vi "Read Configuration Parameters.vi"(8 "error in (no error)":errorcluster, 10 "refnum":T1, 11 "HW Configuration in":refnum<class "HW Configuration.lvclass">) -> (0 "error out":errorcluster, 2 "refnum out":T1, 3 "HW Configuration out":refnum<class "HW Configuration.lvclass">)   [LabVIEW 2017, in "Hardware.lvlib" / "HW Configuration.lvclass"]
uses:
  HW Configuration.lvclass
  C:/Program Files (x86)/National Instruments/LabVIEW 2017/user.lib/Configuration Dialog Actor/Configuration.lvclass
  <vilib>/Utility/config.llb/Config Data RefNum.ctl
  <userlib>/Configuration Dialog Actor/Configuration.lvclass/Configuration.ctl
  HW Configuration.lvclass/HW Configuration.ctl
  <userlib>/Configuration Dialog Actor/Configuration.lvclass
  <vilib>/Utility/config.llb/NI_LVConfig.lvlib
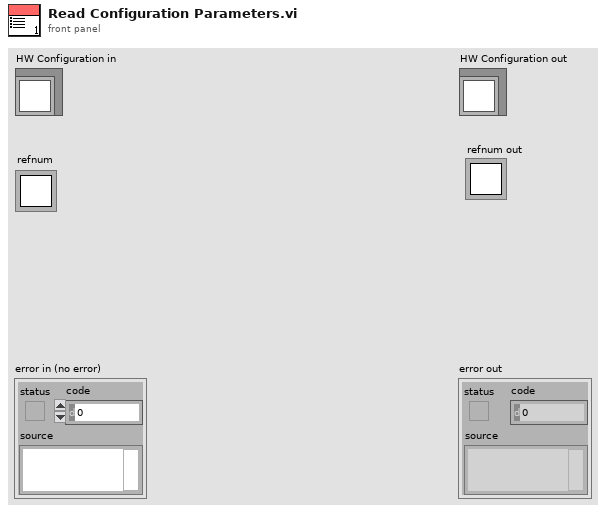
[diagram p1: front panel]
types:
  T1 = typedef "NI_LVConfig.lvlib/Config Data RefNum.ctl" = refnum<k1>
  T2 = cluster{"Device Name":string, "Channel Mapping (Device -> Channel)":string[][]}
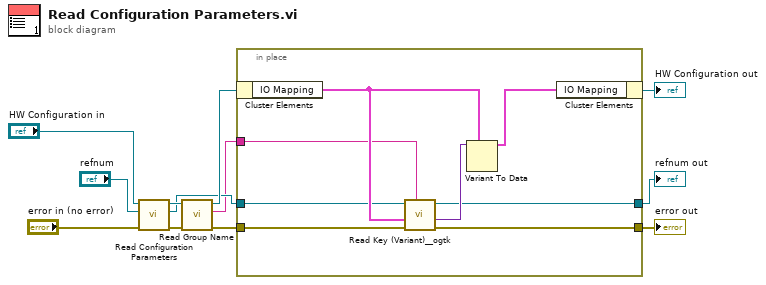
[diagram p0: block diagram]
diagram:
  n1 = call-parent "Read Configuration Parameters.vi"("error in (no error)"="error in (no error)", "refnum"="refnum", "Configuration in"="HW Configuration in") -> ("error out"=w6:errorcluster, "refnum out"=w7:T1, "Configuration out"=w9:refnum<class "HW Configuration.lvclass">)  [unwired: 6 in]
  n2 = call <userlib>:"Read Group Name.vi"("error in (no error)"=w6, "Configuration in"=w9) -> ("error out"=w5:errorcluster, "Group Name"=w4:string, "Configuration out"=w8:refnum<class "HW Configuration.lvclass">)  [unwired: 7 in]
  n3 = in-place {
    in-place-border: w7 -> [w17]
    in-place-border: [w16] -> w3
    in-place-border: w5 -> [w15]
    in-place-border: [w14] -> w1
    in-place-border: w4 -> [w13]
    n4 = in-place-cluster #1(w8) -> ("IO Mapping"=w20:T2)
    n5 = call <userlib>:"Read Key (Variant)__ogtk.vi"("section"=w13, "error in (no error)"=w15, "type"=w20, "refnum"=w17) -> ("error out"=w14:errorcluster, "key-value"=w19:variant, "refnum out"=w16:T1)  [unwired: 4 in, 1 out]
    n6 = Variant To Data(type=w20, Variant=w19) -> (data=w18:T2)  [unwired: 1 in, 1 out]
    n7 = in-place-cluster #1("IO Mapping"=w18) -> (→"HW Configuration out":refnum<class "HW Configuration.lvclass">)
  }
  "error out" <- w1
  "refnum out" <- w3
